vi "5SecVac.vi"() -> ()   [LabVIEW 2016]
panel:
  out "error out 3":errorcluster
  out "source":string
  in  "error in (no error) 2":errorcluster
  out "Array 2":bool[](array[boolean])
  out "error out":errorcluster
  in  "error in (no error)":errorcluster
  out "Array":bool[](array[boolean])
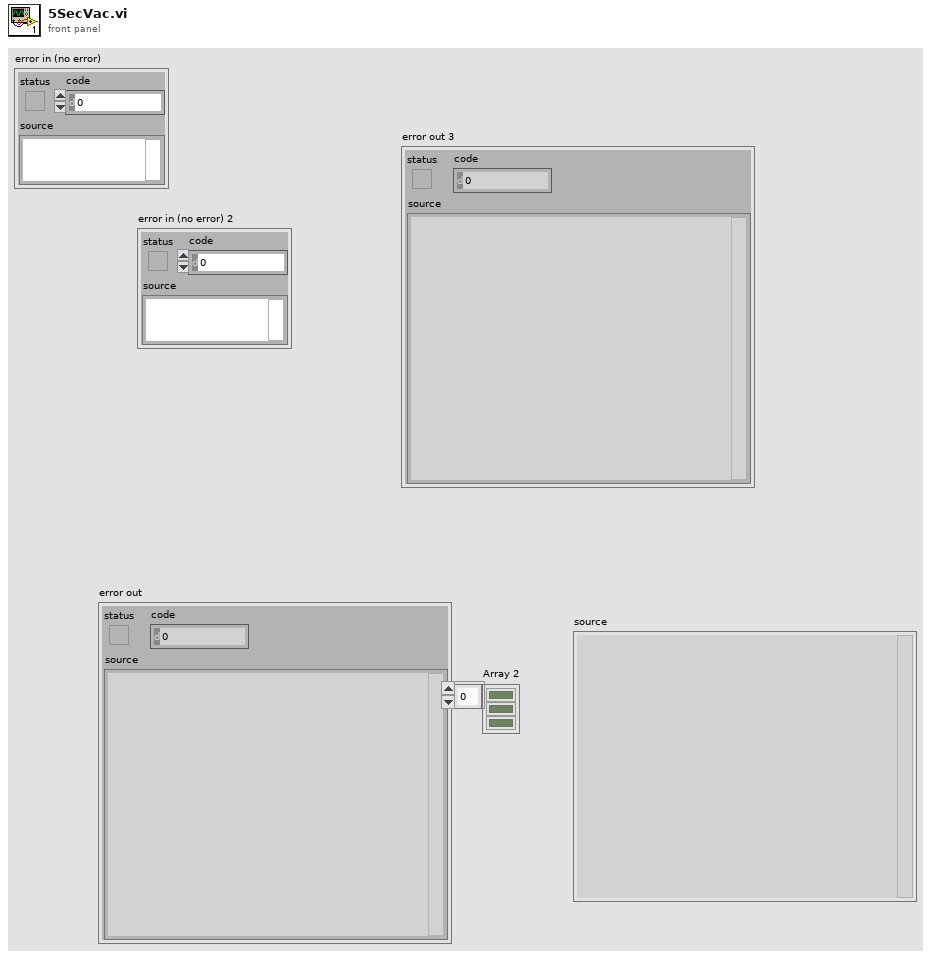
[diagram p1: front panel]
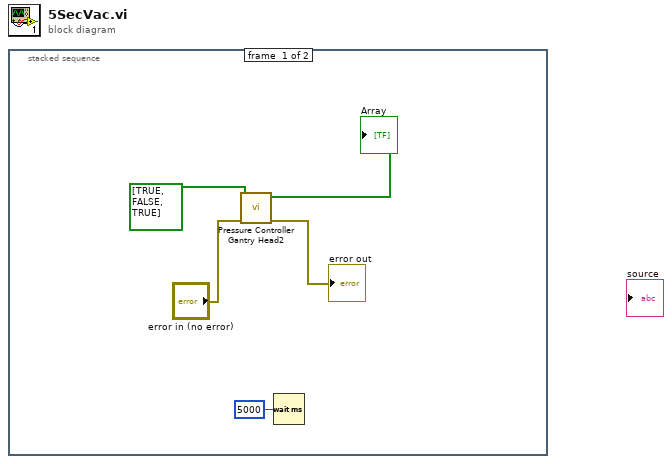
[diagram p0: block diagram]
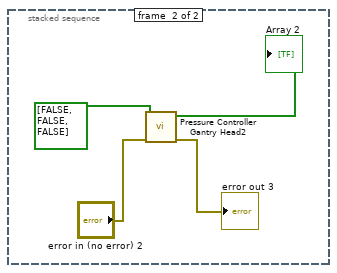
[diagram p2: hidden frame]
diagram:
  n1 = stacked-sequence {
    frame #0 {
      n2 = call "Pressure Controller Gantry Head2.vi"("error in (no error)"="error in (no error)", "data"=bool[] [TRUE, FALSE, TRUE]) -> ("error out"=→"error out":errorcluster, "Output status of pressure lines"=→"Array":bool[])  [unwired: 8 in]
      n3 = Wait (ms)(milliseconds to wait=u32 5000) -> ()  [unwired: 1 out]
    }
    frame #1 {
      n4 = call "Pressure Controller Gantry Head2.vi"("error in (no error)"="error in (no error) 2", "data"=bool[] [FALSE, FALSE, FALSE]) -> ("error out"=→"error out 3":errorcluster, "Output status of pressure lines"=→"Array 2":bool[])  [unwired: 8 in]
    }
  }
